vi "Store.vi"(8 "error in (no error)":errorcluster, 9 "File Name ()":string, 10 "Data Type (0: Entire Instrument State)":u16(ring) items=["Entire Instrument State", "Formatted Data Array", "Image On The LCD Display", "Segment Sweep Table", "Limit Table", "Power Sensor A", "Power Sensor B", "VBA Project", "Loss Compensation Table 1", "Loss Compensation Table 2", "Loss Compensation Table 3", "Loss Compensation Table 4", "Ripple Limit Table"], 11 "VISA resource name":refnum<visa-resource-name>) -> (0 "error out":errorcluster, 3 "VISA resource name out":refnum<visa-resource-name>)   [LabVIEW 2018, in "Agilent ENA Series.lvlib"]
doc: "Saves the specified instrument data into a file."
uses:
  Agilent ENA Series.lvlib
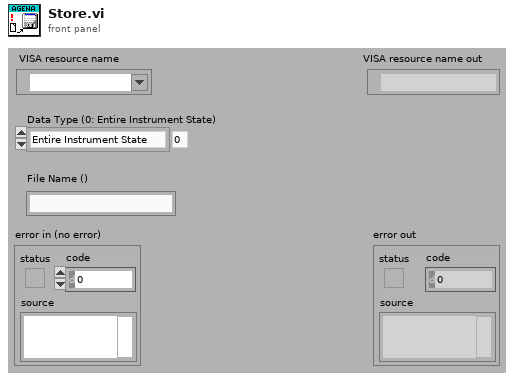
[diagram p1: front panel]
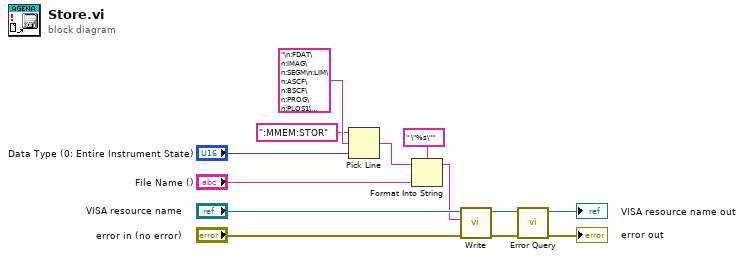
[diagram p0: block diagram]
diagram:
  n1 = Pick Line(string ("")=":MMEM:STOR", multi-line string="\n:FDAT\n:IMAG\n:SEGM\n:LIM\n:ASCF\n:BSCF\n:PROG\n:PLOS1\n:PLOS2\n:PLOS3\n:PLOS4\n:RLIM", line index="Data Type (0: Entire Instrument State)") -> (output string=w6:string)
  n2 = Format Into String(format string=" \"%s\"", initial string=w6, "File Name ()") -> (resulting string=w10:string)  [unwired: 1 in, 1 out]
  n3 = call "Write.vi"("error in (no error)"="error in (no error)", "String ()"=w10, "VISA resource name"="VISA resource name") -> ("error out"=w3:errorcluster, "VISA resource name out"=w4:refnum<visa-resource-name>)  [unwired: 6 in, 1 out]
  n4 = call "Error Query.vi"("error in (no error)"=w3, "VISA resource name"=w4) -> ("error out"=→"error out":errorcluster, "VISA resource name out"=→"VISA resource name out":refnum<visa-resource-name>)  [unwired: 6 in, 2 out]
